vi "pulse_measure_resistance.vi"() -> ()   [LabVIEW 2023]
uses:
  <instrlib>/Keithley 24XX/Public/Data/Read (Single Point).vi
  <vilib>/Utility/file.llb/Write Delimited Spreadsheet (DBL).vi
  <instrlib>/Keithley 24XX/Keithley 24XX.lvlib
  <instrlib>/Tektronix AFG 1000 Series/Tektronix AFG 1000 Series.lvlib
panel:
  in  "save file?":bool
  in  "Path":path
  out "Resistance 2":sgl
  out "applied V 2":dbl
  in  "ampllitude difference":dbl
  out "applied V":dbl
  out "R_V":cluster{dbl[], sgl[]}(graph)
  out "Resistance":sgl
  in  "DC Offset (0.00 V)":dbl
  in  "pulse width(us)":dbl
  in  "Amplitude(1 Vpp)":dbl
  in  "Duty Cycle (%)":dbl=50.0
  in  "Channel (1: Channel 1)":u16(ring)=1 items=["Channel 1"=1, "Channel 2"=2]
  in  "VISA resource name 2":refnum<visa-resource-name>="GPIB0::15::INSTR"
  in  "Current Range":i32(ring) items=["mA"=3, "uA"=6, "nA"=9, "pA"=12]
  in  "milliseconds to wait":u32=10
  in  "VISA resource name":refnum<visa-resource-name>="GPIB0::15::INSTR"
  in  "Keithley Serial Configuration":T1={"Baud Rate"=9600, "Parity"=0, "Data Bits"=8, "Stop Bits"=10, "Flow Control"=0} {"Flow Control" items=["None", "XON/XOFF", "RTS/CTS", "XON/XOFF & RTS/CTS", "DTR/DSR", "XON/XOFF & DTR/DSR"]; "Stop Bits" items=["1.0"=10, "1.5"=15, "2.0"=20]; "Data Bits" items=["7"=7, "8"=8]; "Parity" items=["None", "Odd", "Even", "Mark", "Space"]; "Baud Rate" items=["300"=300, "600"=600, "1200"=1200, "2400"=2400, "4800"=4800, "9600"=9600, "19200"=19200]}
  # "Keithley Setting"
  # "AFG1022 Setting"
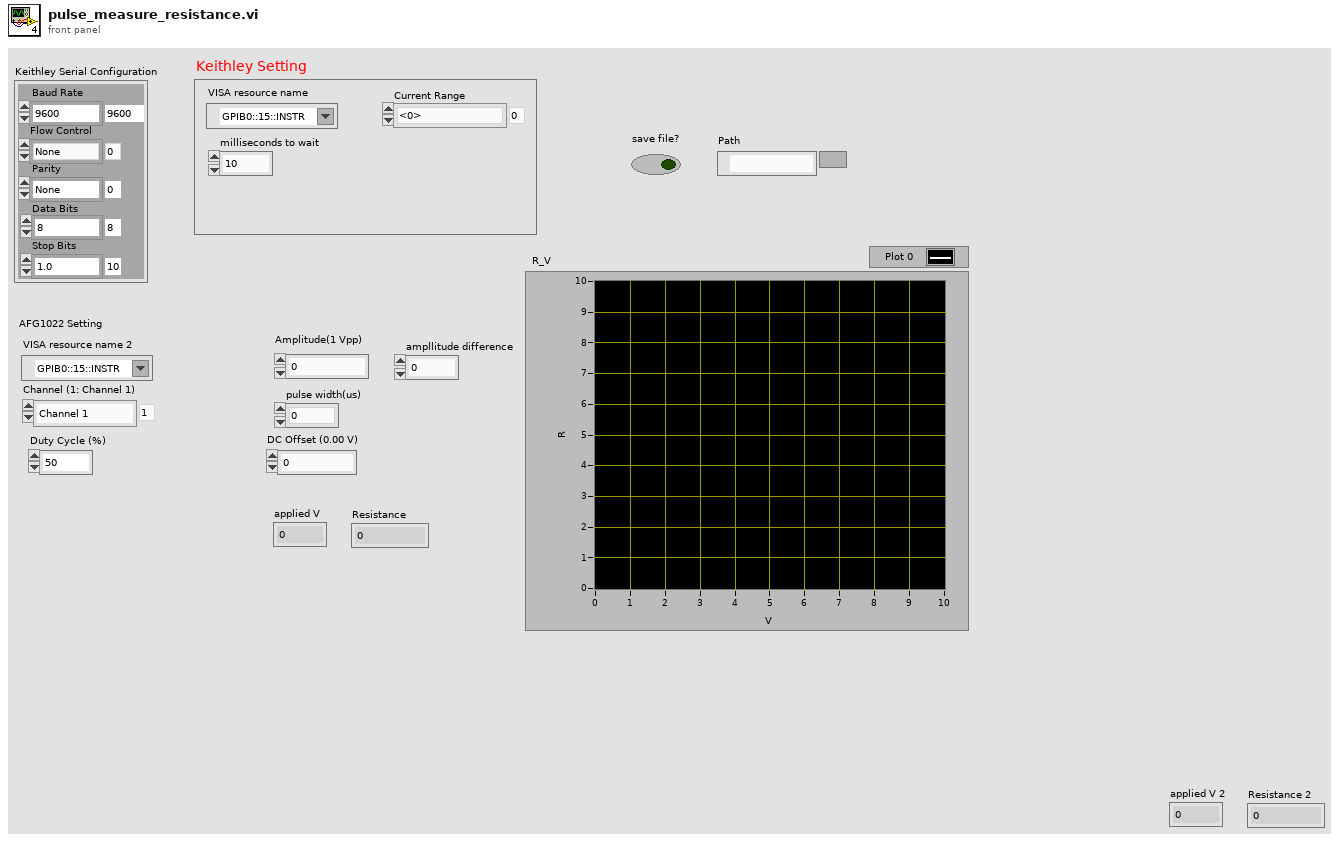
[diagram p1: front panel]
types:
  T1 = cluster{"Baud Rate":u32, "Parity":u16, "Data Bits":u16, "Stop Bits":u16, "Flow Control":u16}
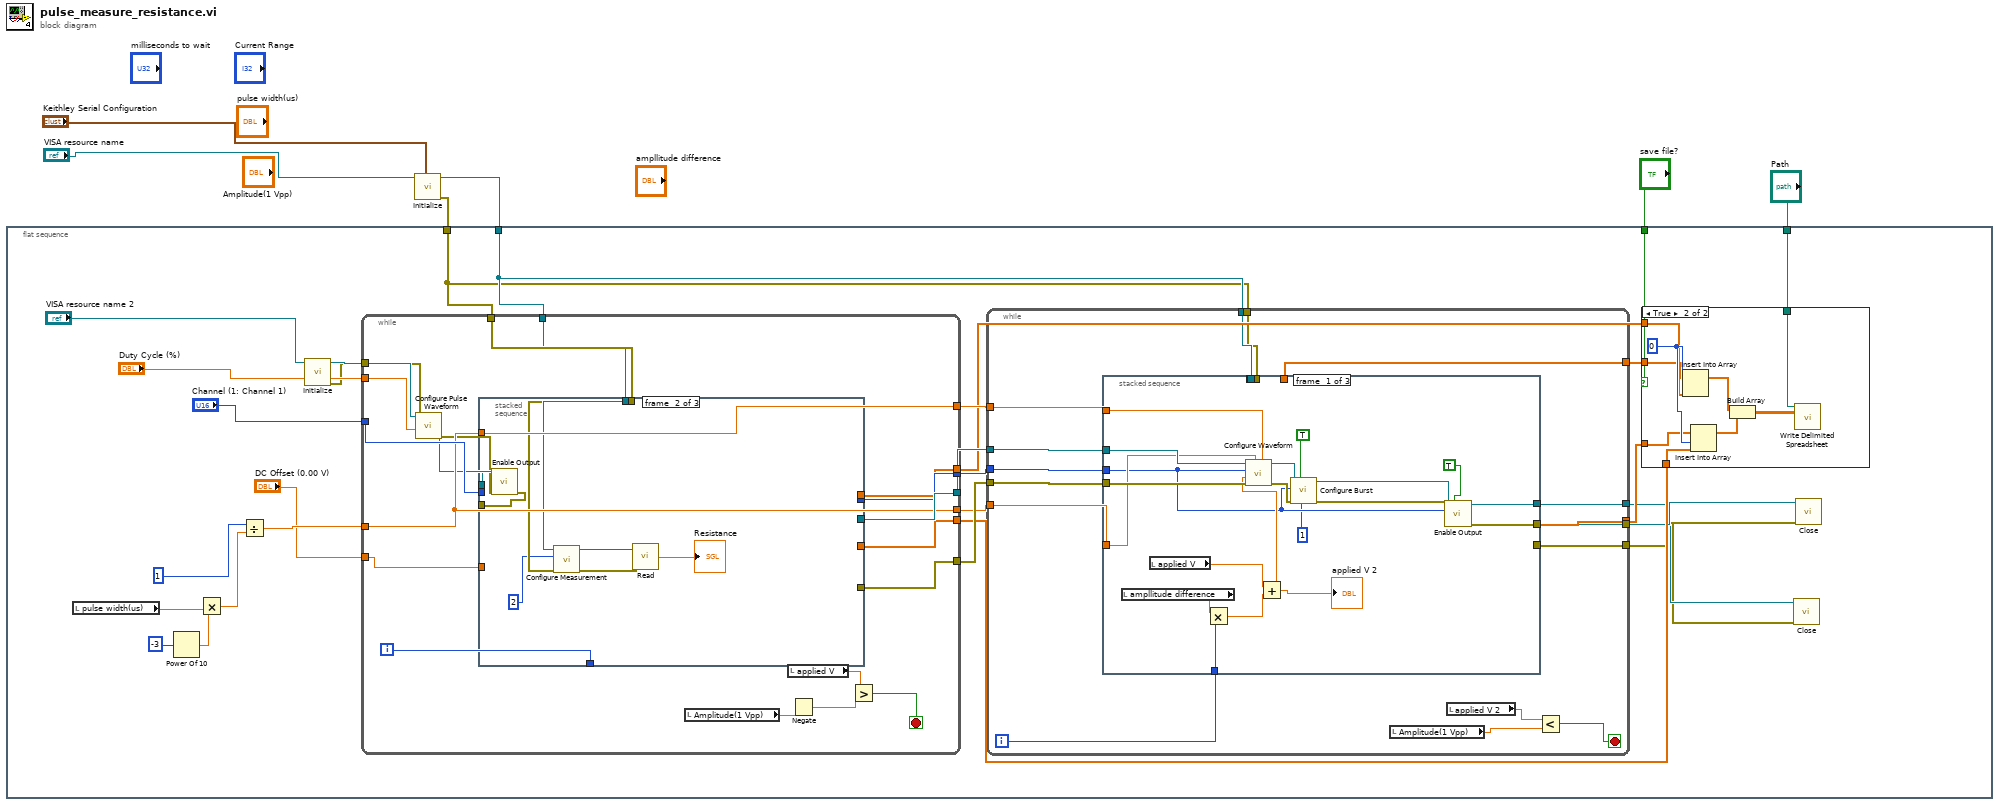
[diagram p0: block diagram]
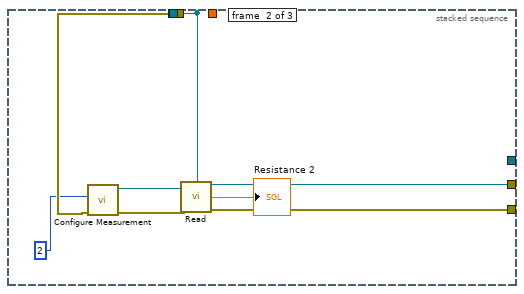
[diagram p3: hidden frame]
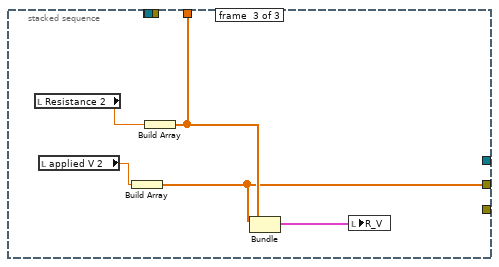
[diagram p4: hidden frame]
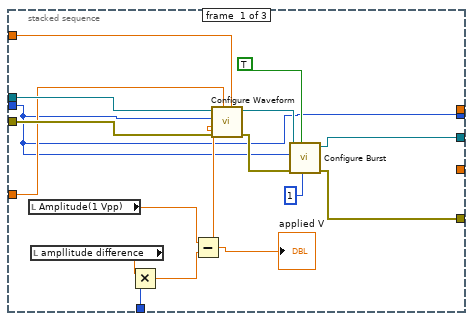
[diagram p5: hidden frame]
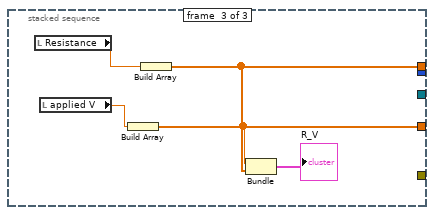
[diagram p6: hidden frame]
diagram:
  n1 = flat-sequence {
    tunnel: w4 -> [w17]
    tunnel: w3 -> [w18]
    tunnel: "save file?" -> [w12]
    tunnel: "Path" -> [w11]
    frame #0 {
      n2 = local read "pulse width(us)"() -> (w30:dbl)
      n3 = Power Of 10(x=-3) -> (10^x=w29:dbl)
      n4 = Multiply(x=w30, y=w29) -> (x*y=w28:dbl)
      n5 = Divide(x=1, y=w28) -> (x/y=w33:dbl)
      n6 = call <instrlib>:"Initialize.vi"("VISA resource name"="VISA resource name 2") -> ("error out"=w24:errorcluster, "VISA resource name out"=w25:refnum<visa-resource-name>)  [unwired: 9 in]
      n7 = while {
        tunnel: "Channel (1: Channel 1)" -> [w115]
        tunnel: w33 -> [w100]
        tunnel: "DC Offset (0.00 V)" -> [w114]
        tunnel: "Duty Cycle (%)" -> [w113]
        tunnel: w17 -> [w112]
        tunnel: w18 -> [w111]
        tunnel: w25 -> [w110]
        tunnel: w24 -> [w109]
        tunnel: [w108] -> w20
        tunnel: [w107] -> w22
        tunnel: [w100] -> w23
        tunnel: [w101] -> w21
        tunnel: [w100] -> w19
        tunnel: [w95] -> w16
        tunnel: [w94] -> w13
        i -> [w106]
        stop <- w102 stop-if-true
        n8 = call <instrlib>:"Configure Pulse Waveform.vi"("error in (no error)"=w109, "Duty Cycle (50%)"=w113, "VISA resource name"=w110) -> ("error out"=w98:errorcluster, "VISA resource name out"=w99:refnum<visa-resource-name>)  [unwired: 7 in]
        n9 = call <instrlib>:"Enable Output.vi"("error in (no error)"=w98, "VISA resource name"=w99) -> ("error out"=w96:errorcluster, "VISA resource name out"=w97:refnum<visa-resource-name>)  [unwired: 8 in]
        n10 = stacked-sequence {
          tunnel: w97 -> [w131 _ _]
          tunnel: w96 -> [w130 _ _]
          tunnel: w115 -> [w117 _ _]
          tunnel: w100 -> [w129 _ _]
          tunnel: w114 -> [w128 _ _]
          tunnel: w111 -> [_ w137 _]
          tunnel: w112 -> [_ w136 _]
          tunnel: [w123 _ _] -> w108
          tunnel: [w124 _ _] -> w107
          tunnel: w106 -> [w121 _ _]
          tunnel: [w117 _ _] -> w101
          tunnel: [_ _ w139] -> w95
          tunnel: [_ _ w138] -> w94
          frame #0 {
            n11 = local read "Amplitude(1 Vpp)"() -> (w120:dbl)
            n12 = local read "ampllitude difference"() -> (w122:dbl)
            n13 = Multiply(x=w122, y=w121) -> (x*y=w119:dbl)
            n14 = Subtract(x=w120, y=w119) -> (x-y=w118:dbl)
            "applied V" <- w118
            n15 = call <instrlib>:"Configure Waveform.vi"("Frequency (1000 Hz)"=w129, "DC Offset (0.00 V)"=w128, "error in (no error)"=w130, "Amplitude (1 Vpp)"=w118, "Channel (1 Channel 1)"=w117, "VISA resource name"=w131) -> ("error out"=w126:errorcluster, "VISA resource name out"=w127:refnum<visa-resource-name>)  [unwired: 4 in]
            n16 = call <instrlib>:"Configure Burst.vi"("Burst Count (1)"=1, "Enable Burst (T: Enable)"=TRUE, "error in (no error)"=w126, "Channel (1 Channel 1)"=w117, "VISA resource name"=w127) -> ("error out"=w123:errorcluster, "VISA resource name out"=w124:refnum<visa-resource-name>)  [unwired: 5 in]
          }
          frame #1 {
            n17 = call <instrlib>:"Configure Measurement.vi"("error in (no error)"=w136, "Function (0: Volts)"=2, "VISA resource name"=w137) -> ("error out"=w133:errorcluster, "VISA resource name out"=w134:refnum<visa-resource-name>)  [unwired: 7 in]
            n18 = call-poly <instrlib>:"Read.vi"("VISA resource name"=w134, "error in (no error)"=w133) -> ("Resistance"=→"Resistance":sgl)  [unwired: 7 in, 6 out]
          }
          frame #2 {
            n19 = local read "Resistance"() -> (w142:sgl)
            n20 = local read "applied V"() -> (w141:dbl)
            n21 = Build Array(w141) -> (w138:dbl[])
            n22 = Build Array(w142) -> (w139:sgl[])
            n23 = Bundle(w138, w139) -> (→"R_V":cluster{dbl[], sgl[]})  [unwired: 1 in]
          }
        }
        n24 = local read "Amplitude(1 Vpp)"() -> (w105:dbl)
        n25 = local read "applied V"() -> (w103:dbl)
        n26 = Negate(x=w105) -> (-x=w104:dbl)
        n27 = Greater?(x=w103, y=w104) -> (0:w102:bool)
      }
      n28 = while {
        tunnel: w23 -> [w60]
        tunnel: w22 -> [w59]
        tunnel: w21 -> [w58]
        tunnel: w20 -> [w57]
        tunnel: w19 -> [w56]
        tunnel: w18 -> [w55]
        tunnel: w17 -> [w54]
        tunnel: [w50] -> w15
        tunnel: [w49] -> w14
        tunnel: [w48] -> w10
        tunnel: [w47] -> w9
        tunnel: [w46] -> w8
        tunnel: [w45] -> w7
        i -> [w61]
        stop <- w51 stop-if-true
        n29 = stacked-sequence {
          tunnel: w59 -> [w80 _ _]
          tunnel: w57 -> [w79 _ _]
          tunnel: w58 -> [w67 _ _]
          tunnel: w60 -> [w78 _ _]
          tunnel: w56 -> [w77 _ _]
          tunnel: [_ w83 _] -> _
          tunnel: w54 -> [_ w88 _]
          tunnel: w61 -> [w69 _ _]
          tunnel: w55 -> [_ w83 _]
          tunnel: [_ _ w90] -> w50
          tunnel: [_ _ w89] -> w49
          tunnel: [_ w82 _] -> w48
          tunnel: [_ w81 _] -> w47
          tunnel: [w63 _ _] -> w46
          tunnel: [w62 _ _] -> w45
          frame #0 {
            n30 = local read "ampllitude difference"() -> (w73:dbl)
            n31 = local read "applied V"() -> (w72:dbl)
            n32 = Multiply(x=w73, y=w69) -> (x*y=w71:dbl)
            n33 = Add(x=w72, y=w71) -> (x+y=w70:dbl)
            "applied V 2" <- w70
            n34 = call <instrlib>:"Configure Waveform.vi"("Frequency (1000 Hz)"=w78, "DC Offset (0.00 V)"=w77, "error in (no error)"=w79, "Amplitude (1 Vpp)"=w70, "Channel (1 Channel 1)"=w67, "VISA resource name"=w80) -> ("error out"=w75:errorcluster, "VISA resource name out"=w76:refnum<visa-resource-name>)  [unwired: 4 in]
            n35 = call <instrlib>:"Configure Burst.vi"("Burst Count (1)"=1, "Enable Burst (T: Enable)"=TRUE, "error in (no error)"=w75, "Channel (1 Channel 1)"=w67, "VISA resource name"=w76) -> ("error out"=w66:errorcluster, "VISA resource name out"=w65:refnum<visa-resource-name>)  [unwired: 5 in]
            n36 = call <instrlib>:"Enable Output.vi"("Enable Output (T: Enable)"=TRUE, "error in (no error)"=w66, "Channel (1: Channel 1)"=w67, "VISA resource name"=w65) -> ("error out"=w62:errorcluster, "VISA resource name out"=w63:refnum<visa-resource-name>)  [unwired: 6 in]
          }
          frame #1 {
            n37 = call <instrlib>:"Configure Measurement.vi"("error in (no error)"=w88, "Function (0: Volts)"=2, "VISA resource name"=w83) -> ("error out"=w85:errorcluster, "VISA resource name out"=w86:refnum<visa-resource-name>)  [unwired: 7 in]
            n38 = call-poly <instrlib>:"Read.vi"("VISA resource name"=w86, "error in (no error)"=w85) -> ("VISA resource name out"=w82:refnum<visa-resource-name>, "Resistance"=→"Resistance 2":sgl, "error out"=w81:errorcluster)  [unwired: 7 in, 4 out]
          }
          frame #2 {
            n39 = local read "Resistance 2"() -> (w93:sgl)
            n40 = local read "applied V 2"() -> (w92:dbl)
            n41 = Build Array(w92) -> (w89:dbl[])
            n42 = Build Array(w93) -> (w90:sgl[])
            n43 = Bundle(w89, w90) -> (w91:cluster{dbl[], sgl[]})  [unwired: 1 in]
            n44 = local write "R_V"(w91) -> ()
          }
        }
        n45 = local read "Amplitude(1 Vpp)"() -> (w52:dbl)
        n46 = local read "applied V 2"() -> (w53:dbl)
        n47 = Less?(x=w53, y=w52) -> (x < y?=w51:bool)
      }
      n48 = case shown="True" w12 {
        tunnel: w16 -> [_ w43]
        tunnel: w15 -> [_ w42]
        tunnel: w14 -> [_ w41]
        tunnel: w13 -> [_ w40]
        tunnel: w11 -> [_ w37]
        frame False {
        }
        frame True {
          w44 = 0
          n49 = Insert Into Array(array=w42, index=w44, new element=w43) -> (w39:sgl[])
          n50 = Insert Into Array(array=w41, index=w44, new element=w40) -> (w38:dbl[])
          n51 = Build Array(w39, w38) -> (w36:dbl[][])
          n52 = call-poly <vilib>:"Write Delimited Spreadsheet.vi"("file path (dialog if empty)"=w37, "2D data"=w36) -> ()  [unwired: 12 in, 2 out]
        }
      }
      n53 = call <instrlib>:"Close.vi"("error in (no error)"=w7, "VISA resource name"=w8) -> ()  [unwired: 9 in, 1 out]
      n54 = call <instrlib>:"Close.vi"("error in (no error)"=w9, "VISA resource name"=w10) -> ()  [unwired: 9 in, 1 out]
    }
  }
  n55 = call <instrlib>:"Initialize.vi"("Serial Configuration"="Keithley Serial Configuration", "VISA resource name"="VISA resource name") -> ("error out"=w4:errorcluster, "VISA resource name out"=w3:refnum<visa-resource-name>)  [unwired: 8 in]
